vi "Get Current LV Dir.vi"(8 "Error In":errorcluster) -> (0 "Error Out":errorcluster, 3 "This LV Directory":path)   [LabVIEW 2019, in "LMH-Toolbox.lvlib"]
doc: "Get the absolute path of LabVIEW directory for the version of LabVIEW this VI is executed in."
uses:
  <vilib>/MakerHub/Toolbox/LMH-Toolbox.lvlib
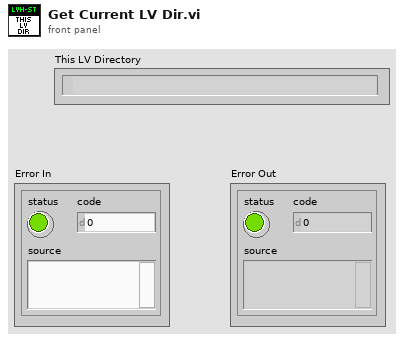
[diagram p1: front panel]
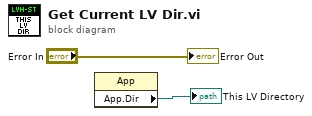
[diagram p0: block diagram]
diagram:
  n1 = property class="App"() -> ("App.Dir"=→"This LV Directory":path)  [unwired: 2 in, 2 out]
  "Error Out" <- "Error In"
